vi "Rectangle Overlay for 2 Cursors.vi"(9 "Radius":cluster{"Rx":sgl, "Ry":sgl}={"Rx"=378.25015, "Ry"=293.73102}, 10 "Coord":cluster{"X":dbl, "Y":dbl}={"X"=5.0, "Y"=5.0}) -> (0 "bottom":dbl, 1 "right":dbl, 2 "Left":dbl, 3 "top":dbl, 4 "Right Bottom":cluster{dbl, dbl}, 5 "Left Top":cluster{dbl, dbl})   [LabVIEW 2013]
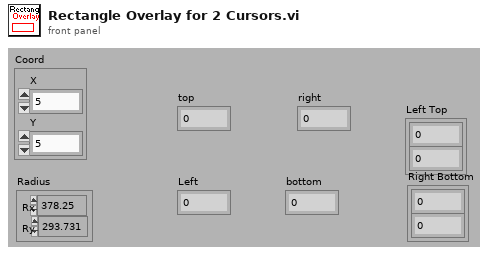
[diagram p1: front panel]
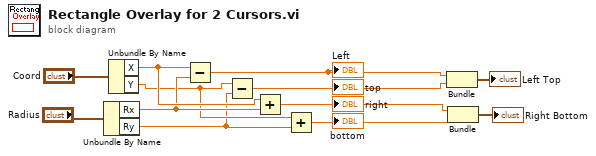
[diagram p0: block diagram]
diagram:
  n1 = Unbundle By Name("Radius") -> ("Rx"=w9:sgl, "Ry"=w7:sgl)
  n2 = Unbundle By Name("Coord") -> ("X"=w10:dbl, "Y"=w8:dbl)
  n3 = Subtract(x=w10, y=w9) -> (x-y=w6:dbl)
  "Left" <- w6
  n4 = Subtract(x=w8, y=w7) -> (x-y=w5:dbl)
  "top" <- w5
  n5 = Add(x=w10, y=w9) -> (x+y=w2:dbl)
  "right" <- w2
  n6 = Add(x=w8, y=w7) -> (x+y=w3:dbl)
  "bottom" <- w3
  n7 = Bundle(w6, w5) -> (→"Left Top":cluster{dbl, dbl})  [unwired: 1 in]
  n8 = Bundle(w2, w3) -> (→"Right Bottom":cluster{dbl, dbl})  [unwired: 1 in]
